vi "Multiplier0.vi"() -> (8 "Multiplier0":refnum<class "Multiplier0.lvclass">)   [LabVIEW 2017, in "Multiplier0.lvclass"]
uses:
  Multiplier0.lvclass
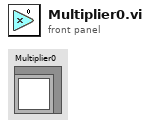
[diagram p1: front panel]
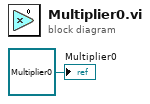
[diagram p0: block diagram]
diagram:
  "Multiplier0" <- refnum<class "Multiplier0.lvclass"> refnum ("Multiplier0.lvclass")
